vi "extract to ROI.vi"(8 "error in (no error)":errorcluster, 9 "Image Dst":T1, 10 "Image":T1, 11 "Thorcam in":refnum<class "Thorcam.lvclass">) -> (0 "error out":errorcluster, 1 "Global Rectangle":i32[](array[numeric]), 2 "Image Out (duplicate)":T1, 3 "Thorcam out":refnum<class "Thorcam.lvclass">)   [LabVIEW 2012, in "Thorcam.lvclass"]
uses:
  Thorcam.lvclass
  <vilib>/vision/Image Controls.llb/IMAQ Image.ctl
  <vilib>/vision/NI_Vision_Development_Module.lvlib
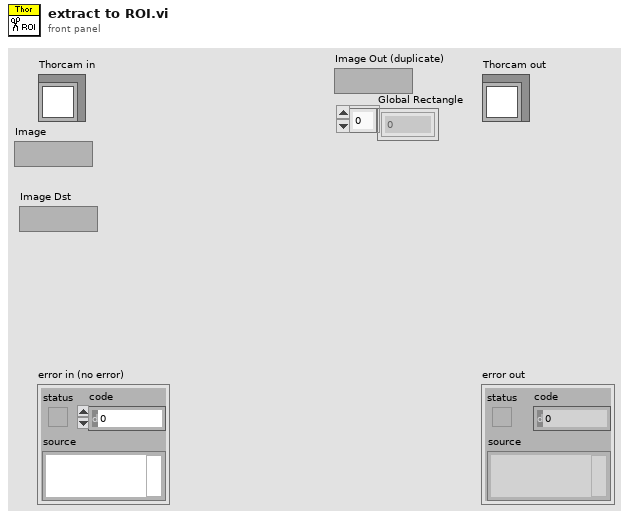
[diagram p1: front panel]
types:
  T1 = typedef "IMAQ Image.ctl" = refnum<image>
  T2 = typedef "ROI Descriptor" = cluster{"Global Rectangle":i32[], "Contours":cluster{"ID":enum32{"External", "Internal"}, "Type":u32, "Coordinates":i32[]}[]}
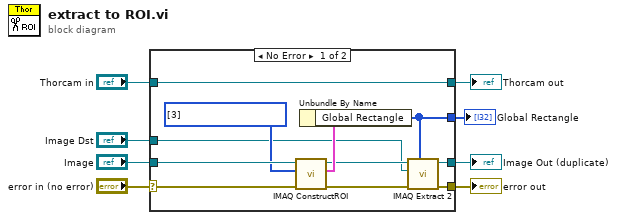
[diagram p0: block diagram]
diagram:
  n1 = case shown="No Error" "error in (no error)" {
    selector: "error in (no error)" -> [w17 w21]
    tunnel: [w13 w21] -> w7
    tunnel: [w19 w20] -> w5
    tunnel: "Thorcam in" -> [w19 w20]
    tunnel: "Image" -> [w18 _]
    tunnel: [w11 _] -> w3
    tunnel: "Image Dst" -> [w10 _]
    tunnel: [w9 _] -> w1
    frame No Error {
      w16 = u32[] [3] items=["No Selection", "Point", "Line", "Rectangle", "Oval", "Polygon", "Freehand Region", "Annulus", "Zoom", "Pan", "Broken Line", "Freehand Line", "Rotated Rectangle"] ("Tools")
      n2 = call "IMAQ ConstructROI"("error in (no error)"=w17, "Tools"=w16, "Image"=w18) -> ("error out"=w14:errorcluster, "ROI Descriptor Out"=w15:T2, "Image Out (duplicate)"=w12:T1)  [unwired: 5 in, 1 out]
      n3 = Unbundle By Name(w15) -> ("Global Rectangle"=w9:i32[])
      n4 = call "IMAQ Extract 2"("Optional Rectangle"=w9, "error in (no error)"=w14, "Image Dst"=w10, "Image Src"=w12) -> ("error out"=w13:errorcluster, "Image Dst Out"=w11:T1)  [unwired: 6 in]
    }
    frame Error {
    }
  }
  "error out" <- w7
  "Thorcam out" <- w5
  "Image Out (duplicate)" <- w3
  "Global Rectangle" <- w1
